vi "量測_VI_Offect2.vi"(0 "Image":T1, 1 "pixel轉mm":dbl, 5 "data":cluster{sgl, sgl}, 7 "圓心 (Pixels)":cluster{"X":sgl, "Y":sgl}, 9 "左邊座標":T2, 11 "右邊座標":T2, 12 "offect總值 in":cluster{"總值左in":dbl, "總值右in":dbl}) -> (4 "左X分量":dbl, 6 "左Y分量":dbl, 8 "右X分量":dbl, 10 "右Y分量":dbl, 15 "offect總值 out":cluster{"總值左out":dbl, "總值右out ":dbl})   [LabVIEW 2015]
uses:
  <vilib>/vision/Image Controls.llb/IMAQ Image.ctl
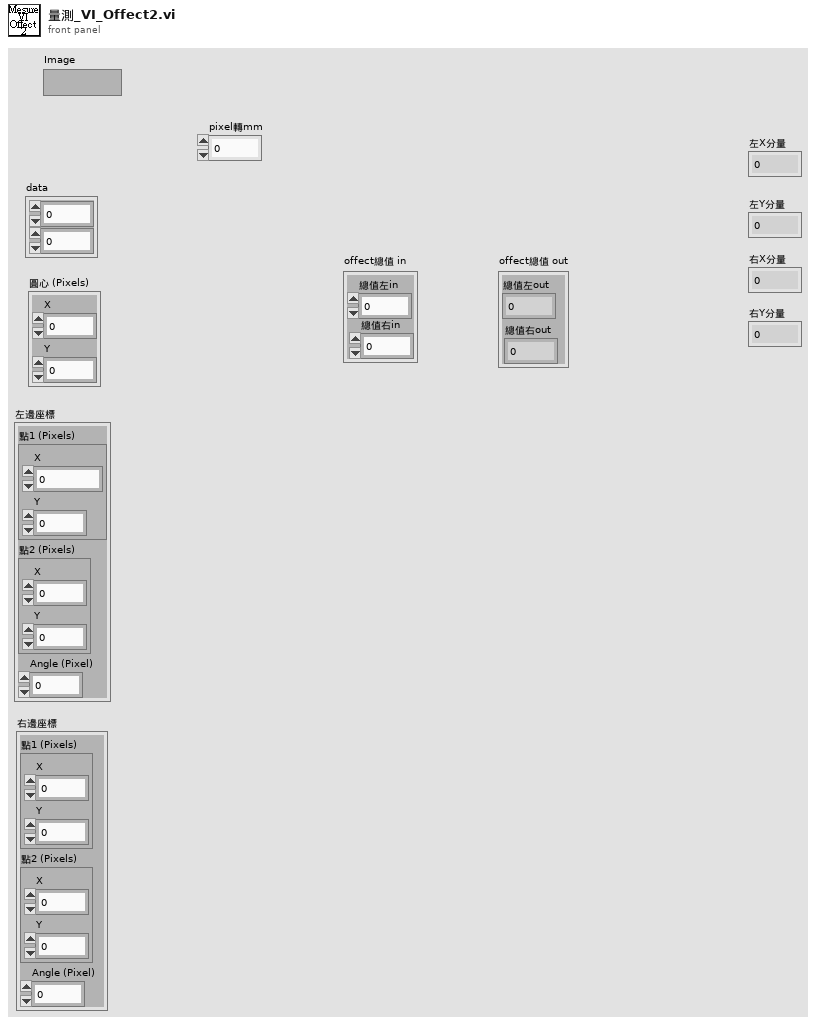
[diagram p1: front panel]
types:
  T1 = typedef "IMAQ Image.ctl" = refnum<image>
  T2 = cluster{"點1 (Pixels)":cluster{"X":sgl, "Y":sgl}, "點2 (Pixels)":cluster{"X":sgl, "Y":sgl}, "Angle (Pixel)":dbl}
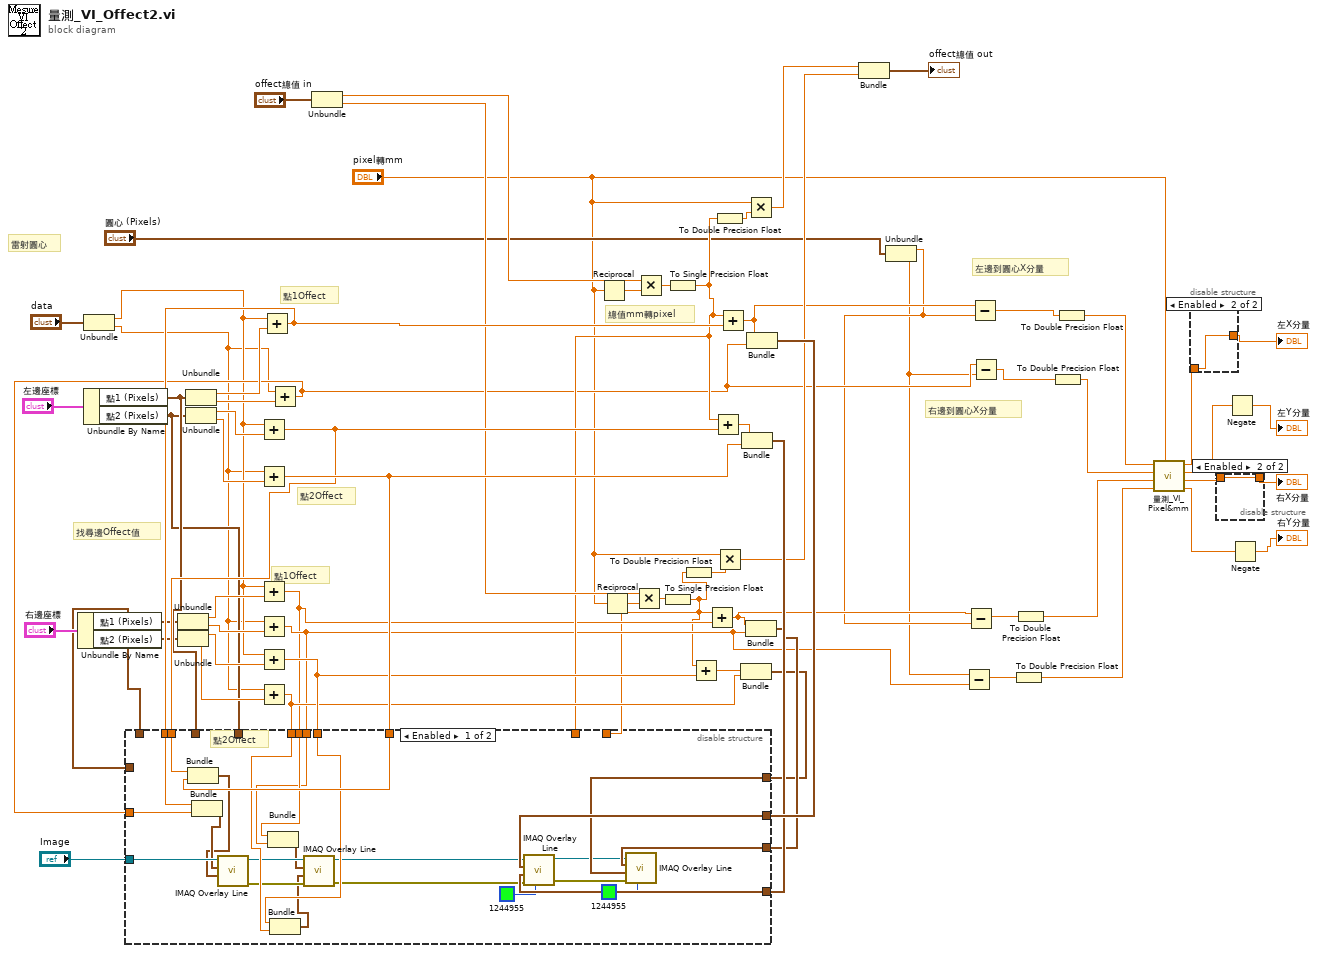
[diagram p0: block diagram]
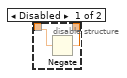
[diagram p2: hidden frame]
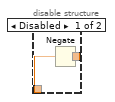
[diagram p3: hidden frame]
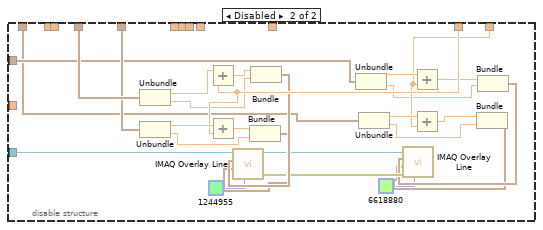
[diagram p4: hidden frame]
diagram:
  # "右邊到圓心X分量"
  # "左邊到圓心X分量"
  # "雷射圓心"
  # "總值mm轉pixel"
  # "點1Offect"
  # "點2Offect"
  # "點1Offect"
  # "找尋邊Offect值"
  n1 = Unbundle By Name("右邊座標") -> ("點1 (Pixels)"=w30:cluster{"X":sgl, "Y":sgl}, "點2 (Pixels)"=w29:cluster{"X":sgl, "Y":sgl})
  n2 = Unbundle("data") -> (w10:sgl, w9:sgl)
  n3 = Unbundle By Name("左邊座標") -> ("點1 (Pixels)"=w33:cluster{"X":sgl, "Y":sgl}, "點2 (Pixels)"=w32:cluster{"X":sgl, "Y":sgl})
  n4 = Unbundle(w30) -> ("X"=w62:sgl, "Y"=w61:sgl)
  n5 = Unbundle(w29) -> ("X"=w60:sgl, "Y"=w59:sgl)
  n6 = Unbundle(w33) -> ("X"=w66:sgl, "Y"=w65:sgl)
  n7 = Unbundle(w32) -> ("X"=w64:sgl, "Y"=w63:sgl)
  n8 = Add(x=w10, y=w64) -> (x+y=w53:sgl)
  n9 = Add(x=w9, y=w63) -> (x+y=w55:sgl)
  n10 = Add(x=w10, y=w62) -> (x+y=w12:sgl)
  n11 = Add(x=w9, y=w61) -> (x+y=w13:sgl)
  n12 = Add(x=w10, y=w60) -> (x+y=w45:sgl)
  n13 = Add(x=w9, y=w59) -> (x+y=w43:sgl)
  n14 = Add(x=w10, y=w66) -> (x+y=w56:sgl)
  n15 = Add(x=w9, y=w65) -> (x+y=w25:sgl)
  n16 = Unbundle("offect總值 in") -> ("總值左in"=w49:dbl, "總值右in"=w47:dbl)
  n17 = Reciprocal(x="pixel轉mm") -> (1/x=w50:dbl)
  n18 = Reciprocal(x="pixel轉mm") -> (1/x=w48:dbl)
  n19 = Multiply(x=w47, y=w48) -> (x*y=w46:dbl)
  n20 = Multiply(x=w49, y=w50) -> (x*y=w51:dbl)
  n21 = To Single Precision Float(number=w46) -> (single precision float=w11:sgl)
  n22 = To Single Precision Float(number=w51) -> (single precision float=w31:sgl)
  n23 = To Double Precision Float(number=w11) -> (double precision float=w38:dbl)
  n24 = Add(x=w11, y=w45) -> (x+y=w44:sgl)
  n25 = Add(x=w11, y=w12) -> (x+y=w23:sgl)
  n26 = Add(x=w31, y=w53) -> (x+y=w54:sgl)
  n27 = To Double Precision Float(number=w31) -> (double precision float=w39:dbl)
  n28 = Multiply(x="pixel轉mm", y=w38) -> (x*y=w36:dbl)
  n29 = Add(x=w31, y=w56) -> (x+y=w27:sgl)
  n30 = Bundle(w44, w43) -> (w41:cluster{sgl, sgl})  [unwired: 1 in]
  n31 = Bundle(w54, w55) -> (w52:cluster{sgl, sgl})  [unwired: 1 in]
  n32 = Multiply(x="pixel轉mm", y=w39) -> (x*y=w37:dbl)
  n33 = Bundle(w23, w13) -> (w42:cluster{sgl, sgl})  [unwired: 1 in]
  n34 = Bundle(w27, w25) -> (w57:cluster{sgl, sgl})  [unwired: 1 in]
  n35 = disable-structure shown="Enabled" {
    disable-tunnel: w57 -> [w93 _]
    disable-tunnel: w56 -> [w92 _]
    disable-tunnel: w55 -> [w91 _]
    disable-tunnel: w53 -> [w90 _]
    disable-tunnel: w52 -> [w89 _]
    disable-tunnel: w25 -> [w88 _]
    disable-tunnel: w12 -> [w87 _]
    disable-tunnel: w13 -> [w86 _]
    disable-tunnel: w45 -> [w85 _]
    disable-tunnel: w43 -> [w84 _]
    disable-tunnel: w42 -> [w83 _]
    disable-tunnel: w41 -> [w82 _]
    disable-tunnel: "Image" -> [w81 w120]
    disable-tunnel: w33 -> [_ w119]
    disable-tunnel: w32 -> [_ w118]
    disable-tunnel: w31 -> [_ w115]
    disable-tunnel: w30 -> [_ w106]
    disable-tunnel: w29 -> [_ w105]
    disable-tunnel: w11 -> [_ w102]
    frame Enabled {
      # "點2Offect"
      n36 = Bundle(w90, w91) -> (w79:cluster{sgl, sgl})  [unwired: 1 in]
      n37 = Bundle(w92, w88) -> (w80:cluster{sgl, sgl})  [unwired: 1 in]
      n38 = call "IMAQ Overlay Line"("End Point"=w79, "Start Point"=w80, "Image"=w81) -> ("error out"=w77:errorcluster, "Image Out"=w78:T1)  [unwired: 7 in]
      n39 = Bundle(w87, w86) -> (w76:cluster{sgl, sgl})  [unwired: 1 in]
      n40 = Bundle(w85, w84) -> (w69:cluster{sgl, sgl})  [unwired: 1 in]
      n41 = call "IMAQ Overlay Line"("error in (no error)"=w77, "End Point"=w69, "Start Point"=w76, "Image"=w78) -> ("error out"=w74:errorcluster, "Image Out"=w75:T1)  [unwired: 6 in]
      n42 = call "IMAQ Overlay Line"("Color"=u32 1244955, "error in (no error)"=w74, "End Point"=w89, "Start Point"=w93, "Image"=w75) -> ("error out"=w72:errorcluster, "Image Out"=w73:T1)  [unwired: 5 in]
      n43 = call "IMAQ Overlay Line"("Color"=u32 1244955, "error in (no error)"=w72, "End Point"=w82, "Start Point"=w83, "Image"=w73) -> ()  [unwired: 5 in, 2 out]
    }
    frame Disabled {
      n44 = Unbundle(w119) -> ("X"=w117:sgl, "Y"=w113:sgl)
      n45 = Unbundle(w118) -> ("X"=w116:sgl, "Y"=w110:sgl)
      n46 = Add(x=w117, y=w115) -> (x+y=w114:sgl)
      n47 = Add(x=w116, y=w115) -> (x+y=w111:sgl)
      n48 = Bundle(w111, "Y"=w110) -> (w109:cluster{sgl, "Y":sgl})  [unwired: 1 in]
      n49 = Bundle(w114, "Y"=w113) -> (w112:cluster{sgl, "Y":sgl})  [unwired: 1 in]
      n50 = call "IMAQ Overlay Line"("Color"=u32 1244955, "End Point"=w109, "Start Point"=w112, "Image"=w120) -> ("error out"=w108:errorcluster, "Image Out"=w107:T1)  [unwired: 6 in]
      n51 = Unbundle(w106) -> ("X"=w104:sgl, "Y"=w100:sgl)
      n52 = Unbundle(w105) -> ("X"=w103:sgl, "Y"=w98:sgl)
      n53 = Add(x=w104, y=w102) -> (x+y=w101:sgl)
      n54 = Add(x=w103, y=w102) -> (x+y=w99:sgl)
      n55 = Bundle(w99, "Y"=w98) -> (w96:cluster{sgl, "Y":sgl})  [unwired: 1 in]
      n56 = Bundle(w101, "Y"=w100) -> (w97:cluster{sgl, "Y":sgl})  [unwired: 1 in]
      n57 = call "IMAQ Overlay Line"("Color"=u32 6618880, "error in (no error)"=w108, "End Point"=w96, "Start Point"=w97, "Image"=w107) -> ()  [unwired: 5 in, 2 out]
    }
  }
  n58 = Bundle(w37, w36) -> (→"offect總值 out":cluster{dbl, dbl})  [unwired: 1 in]
  n59 = Unbundle("圓心 (Pixels)") -> ("X"=w22:sgl, "Y"=w19:sgl)
  n60 = Subtract(x=w19, y=w13) -> (x-y=w20:sgl)
  n61 = Subtract(x=w23, y=w22) -> (x-y=w21:sgl)
  n62 = Subtract(x=w27, y=w22) -> (x-y=w26:sgl)
  n63 = Subtract(x=w25, y=w19) -> (x-y=w24:sgl)
  n64 = To Double Precision Float(number=w20) -> (double precision float=w15:dbl)
  n65 = To Double Precision Float(number=w21) -> (double precision float=w16:dbl)
  n66 = To Double Precision Float(number=w24) -> (double precision float=w17:dbl)
  n67 = To Double Precision Float(number=w26) -> (double precision float=w18:dbl)
  n68 = call "量測_VI_Pixel&mm.vi"("Pixel轉mm"="pixel轉mm", "Distance右垂直(pixel)"=w15, "Distances右水平(pixel)"=w16, "Distance左垂直(pixel)"=w17, "Distances左水平(pixel)"=w18) -> ("Distance右垂直(mm)"=w2:dbl, "Distances右水平(mm)"=w6:dbl, "Distance左垂直(mm)"=w4:dbl, "Distances左水平(mm)"=w8:dbl)  [unwired: 3 in]
  n69 = disable-structure shown="Enabled" {
    disable-tunnel: w8 -> [w122 w123]
    disable-tunnel: [w121 w123] -> w7
    frame Disabled {
      n70 = Negate(x=w122) -> (-x=w121:dbl)
    }
    frame Enabled {
    }
  }
  "左X分量" <- w7
  n71 = disable-structure shown="Enabled" {
    disable-tunnel: w6 -> [w125 w126]
    disable-tunnel: [w124 w126] -> w5
    frame Disabled {
      n72 = Negate(x=w125) -> (-x=w124:dbl)
    }
    frame Enabled {
    }
  }
  "右X分量" <- w5
  n73 = Negate(x=w4) -> (-x=→"左Y分量":dbl)
  n74 = Negate(x=w2) -> (-x=→"右Y分量":dbl)
